vi "write command.vi"(8 "error in (no error)":errorcluster, 10 "command":T1, 11 "Request in":refnum<class "Request.lvclass">) -> (0 "error out":errorcluster, 3 "Request out":refnum<class "Request.lvclass">)   [LabVIEW 2018, in "Request.lvclass"]
uses:
  Request.lvclass
  Request.lvclass/Request.ctl
  Command/Command.lvclass/Command.ctl
  Command/Command.lvclass
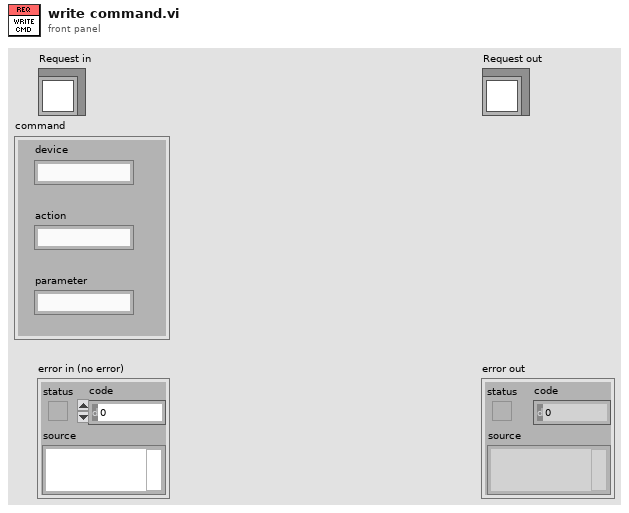
[diagram p1: front panel]
types:
  T1 = cluster{"device":string, "action":string, "parameter":string}
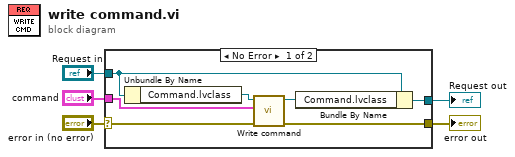
[diagram p0: block diagram]
diagram:
  n1 = case shown="No Error" "error in (no error)" {
    selector: "error in (no error)" -> [w8 w14]
    tunnel: [w7 w14] -> w4
    tunnel: [w11 w13] -> w2
    tunnel: "Request in" -> [w12 w13]
    tunnel: "command" -> [w6 _]
    frame No Error {
      n2 = Unbundle By Name(w12) -> ("Command.lvclass"=w10:refnum<class "Command.lvclass">)
      n3 = call "Write command.vi"("error in (no error)"=w8, "command"=w6, "Command in"=w10) -> ("error out"=w7:errorcluster, "Command out"=w9:refnum<class "Command.lvclass">)  [unwired: 7 in]
      n4 = Bundle By Name(cluster=w12, "Command.lvclass"=w9) -> (w11:refnum<class "Request.lvclass">)
    }
    frame Error {
    }
  }
  "error out" <- w4
  "Request out" <- w2
